vi "Init.vi"(8 "error in (no error)":errorcluster, 10 "Node Reg":refnum<k20>, 11 "Array in":refnum<class "Array.lvclass">) -> (0 "error out":errorcluster, 3 "Array out":refnum<class "Array.lvclass">)   [LabVIEW 2025, in "Array.lvclass"]
uses:
  Array.lvclass
  Node.lvclass
  <vilib>/xml/NI_XML.lvlib
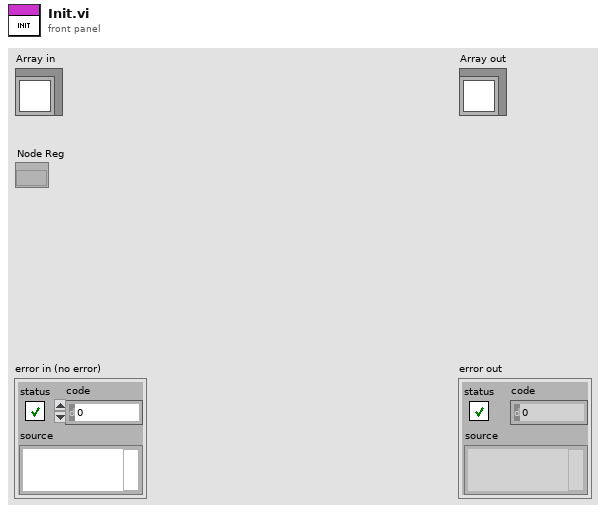
[diagram p1: front panel]
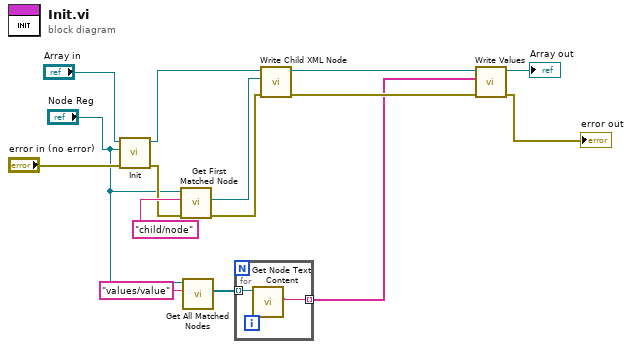
[diagram p0: block diagram]
diagram:
  n1 = call-parent "Init.vi"("error in (no error)"="error in (no error)", "Node Reg"="Node Reg", "Node in"="Array in") -> ("error out"=w9:errorcluster, "Node out"=w15:refnum<class "Array.lvclass">)  [unwired: 7 in]
  n2 = call <vilib>:"Get First Matched Node.vi"("error in (no error)"=w9, "XPath expression"="child/node", "node in"="Node Reg") -> ("error out"=w8:errorcluster, "node result"=w10:refnum<k20>)  [unwired: 6 in, 1 out]
  n3 = call <vilib>:"Get All Matched Nodes.vi"("XPath expression"="values/value", "node in"="Node Reg") -> ("node result array"=w2:refnum<k20>[])  [unwired: 7 in, 2 out]
  n4 = for {
    tunnel: w2 -> [w17] mode=indexing
    tunnel: [w16] -> w1 mode=indexing
    n5 = call <vilib>:"Get Node Text Content.vi"("node in"=w17) -> ("node text"=w16:string)  [unwired: 8 in, 2 out]
  }
  n6 = call-dynamic "Write Child XML Node.vi"("error in (no error)"=w8, "Child XML Node"=w10, "Array in"=w15) -> ("error out"=w6:errorcluster, "Array out"=w12:refnum<class "Array.lvclass">)  [unwired: 7 in]
  n7 = call-dynamic "Write Values.vi"("error in (no error)"=w6, "Values"=w1, "Array in"=w12) -> ("error out"=→"error out":errorcluster, "Array out"=→"Array out":refnum<class "Array.lvclass">)  [unwired: 7 in]
